vi "cDAQ getVolumeInfo.vi"() -> ()   [LabVIEW 2019]
panel:
  out "error out":errorcluster
  out "free (bytes)":i64
  out "size (bytes)":i64
  in  "path":path
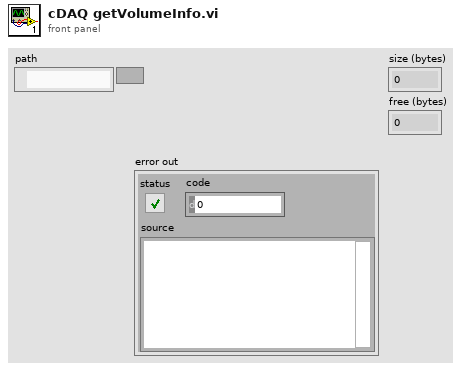
[diagram p1: front panel]
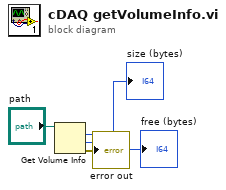
[diagram p0: block diagram]
diagram:
  n1 = Get Volume Info(11:"path") -> (0:→"error out":errorcluster, 1:→"free (bytes)":i64, 2:→"size (bytes)":i64)  [unwired: 1 in, 3 out]
